vi "GlobalDevice.vi"() -> ()   [LabVIEW 2013]
panel:
  in  "ProcessorClockDivider":dbl
  in  "Device Choser":enum32{"Stage", "Mirror"}(radio)
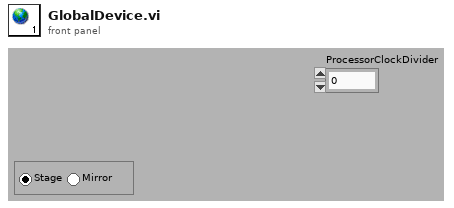
[diagram p1: front panel]
diagram:
